vi "Actor Core.vi"(8 "error in (no error)":errorcluster, 11 "Mediated Asynchronous Actor in":refnum<class "Mediated Asynchronous Actor.lvclass">) -> (0 "error out":errorcluster, 3 "Mediated Asynchronous Actor out":refnum<class "Mediated Asynchronous Actor.lvclass">)   [LabVIEW 2016, in "Stream Mediator.lvlib" / "Mediated Asynchronous Actor.lvclass"]
doc: "--\nCopyright © 2017 Composed SystemsI All rights reserved.\n\nAuthor: Jon McBee <jon.mcbee@composed.io>\n\nThis library is provided \"AS IS\" ,WITHOUT WARRANTIES OR\nCONDITIONS OF ANY KIND, either express or implied.\n\nComposed Systems -- composed.io\n\nStream 0.0.1.1\nJon McBee - Composed Systems\nCopyright (c) 2017, Composed Systems"
uses:
  <userlib>/Composed Systems/Stream/Mediator/Classes/Mediated Asynchronous Actor/Mediated Asynchronous Actor.lvclass
  <userlib>/Composed Systems/Stream/Mediator/Classes/Mediated Asynchronous Actor/Mediated Asynchronous Actor.lvclass/Mediated Asynchronous Actor.ctl
  <userlib>/Composed Systems/Stream/Mediator/Classes/Message Transport Queue/Message Transport Queue.lvclass
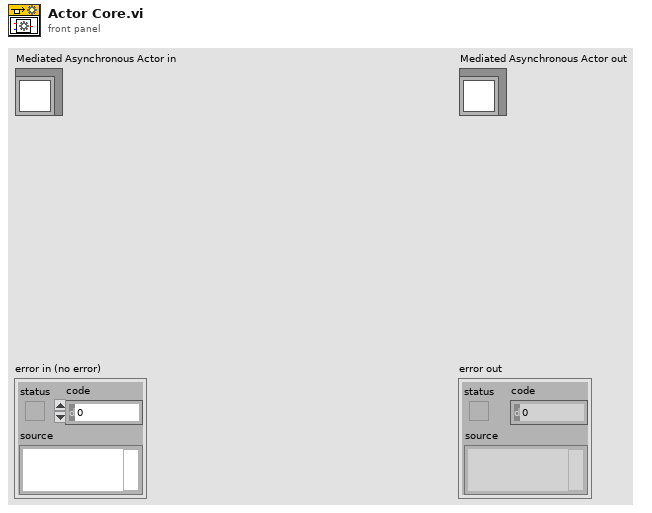
[diagram p1: front panel]
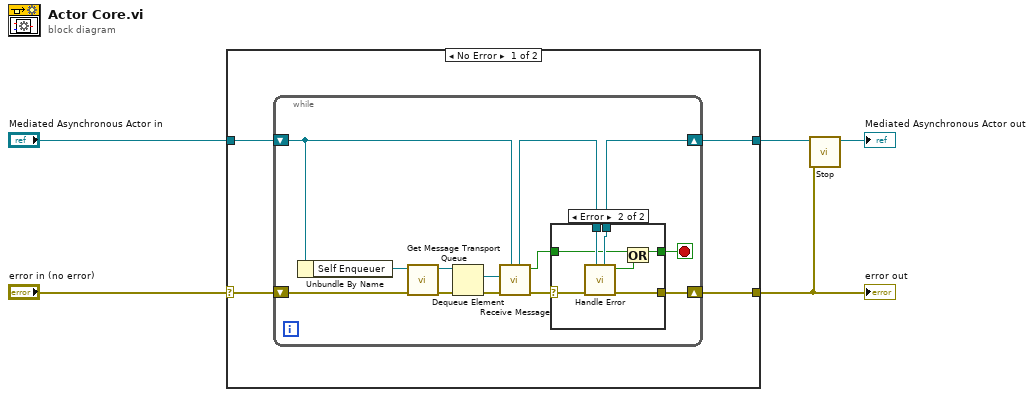
[diagram p0: block diagram]
diagram:
  n1 = case shown="No Error" "error in (no error)" {
    selector: "error in (no error)" -> [w8 w34]
    tunnel: [w6 w34] -> w1
    tunnel: [w7 w33] -> w2
    tunnel: "Mediated Asynchronous Actor in" -> [w9 w33]
    frame No Error {
      n2 = while {
        shift-right: [w12] -> w7
        shift-left: w9 -> [w22]
        shift-right: [w14] -> w6
        shift-left: w8 -> [w19]
        stop <- w10 stop-if-true
        n3 = Unbundle By Name(w22) -> ("Self Enqueuer"=w17:refnum<class "Message Transport Queue.lvclass">)
        n4 = call <userlib>:"Get Message Transport Queue.vi"("error in (no error)"=w19, "Message Transport Queue in"=w17) -> ("error out"=w21:errorcluster, "Queue"=w20:refnum<queue>)  [unwired: 8 in]
        n5 = Dequeue Element(queue=w20, error in (no error)=w21) -> (element=w16:refnum<class "Message Interface.lvclass">, error out=w18:errorcluster)  [unwired: 1 in, 2 out]
        n6 = call-dynamic "Receive Message.vi"("Mediated Asynchronous Actor in"=w22, "error in (no error)"=w18, "Message in"=w16) -> ("error out"=w15:errorcluster, "Stop?"=w11:bool, "Mediated Asynchronous Actor out"=w13:refnum<class "Mediated Asynchronous Actor.lvclass">)  [unwired: 6 in]
        n7 = case shown="Error" w15 {
          selector: w15 -> [w24 w32]
          tunnel: [w24 w31] -> w14
          tunnel: w13 -> [w25 w30]
          tunnel: [w25 w29] -> w12
          tunnel: w11 -> [w23 w28]
          tunnel: [w23 w26] -> w10
          frame No Error {
          }
          frame Error {
            n8 = call-dynamic "Handle Error.vi"("Mediated Asynchronous Actor in"=w30, "error in (no error)"=w32) -> ("error out"=w31:errorcluster, "Stop Actor?"=w27:bool, "Mediated Asynchronous Actor out"=w29:refnum<class "Mediated Asynchronous Actor.lvclass">)  [unwired: 7 in]
            n9 = Or(x=w28, y=w27) -> (x .or. y?=w26:bool)
          }
        }
      }
    }
    frame Error {
    }
  }
  "error out" <- w1
  n10 = call <userlib>:"Stop.vi"("error in (no error)"=w1, "Mediated Asynchronous Actor in"=w2) -> ("Mediated Asynchronous Actor out"=→"Mediated Asynchronous Actor out":refnum<class "Mediated Asynchronous Actor.lvclass">)  [unwired: 9 in]
